vi "Diff Tool.vi"(10 "Reference":string, 11 "Target":string) -> (2 "Highlights":T1(array[cluster]), 3 "Result":string)   [LabVIEW 2020]
uses:
  d41eeba9-a009-4172-b538-d2f3e9e71bd9.vi
  <vilib>/Comparison/Less/Less Functor/Less Functor.lvclass
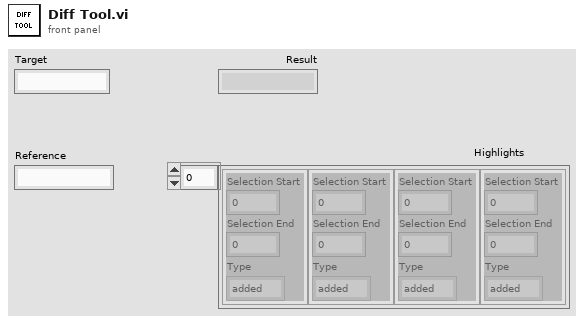
[diagram p1: front panel]
types:
  T1 = cluster{"Selection Start":u32, "Selection End":u32, "Type":enum16{"added", "missing"}}[]
  T2 = cluster{"Selection Start":u32, "Selection End":u32}[]
  T3 = cluster{"Index":i32, "String":string, "Type":enum16{"added", "missing"}}
  T4 = cluster{"Index":i32, "String":string, "Type":enum16{"added", "missing"}}[]
  T5 = cluster{"Selection Start":u32, "Selection End":u32, "Type":enum16{"added", "missing"}}
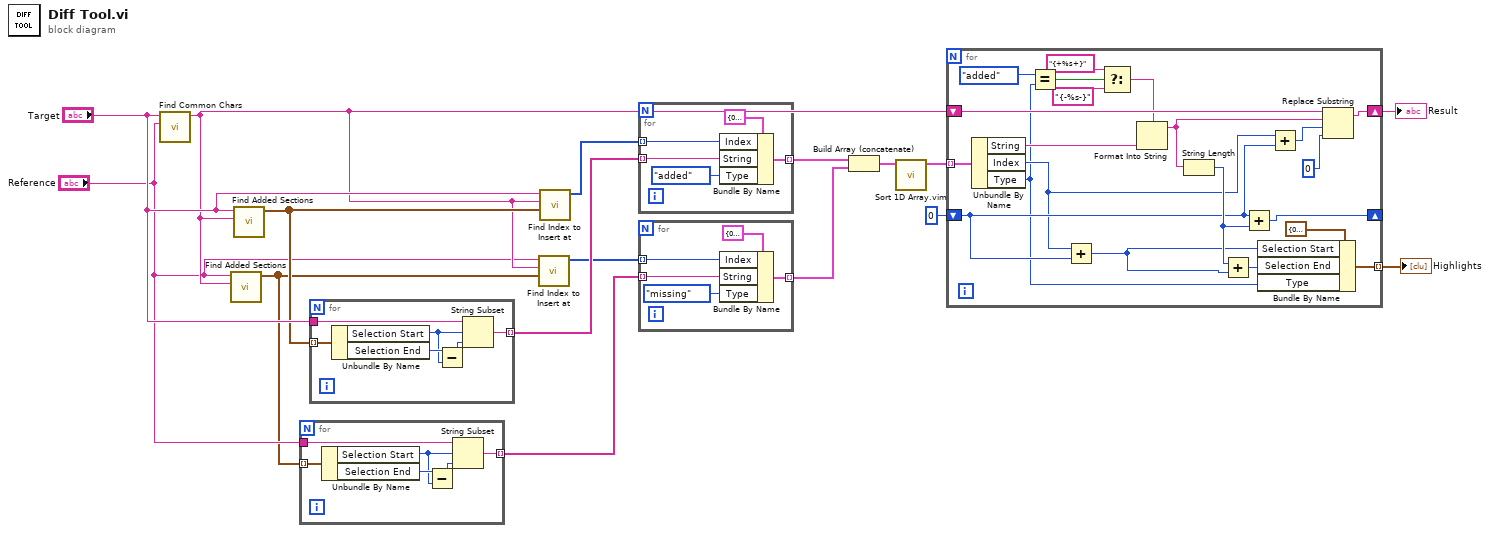
[diagram p0: block diagram]
diagram:
  n1 = call "Find Common Chars.vi"("Reference"="Reference", "Target"="Target") -> ("Common"=w13:string)  [unwired: 9 in]
  n2 = call "Find Added Sections.vi"("Reference"=w13, "Target"="Reference") -> ("Sections in Target"=w11:T2)  [unwired: 9 in]
  n3 = call "Find Added Sections.vi"("Reference"=w13, "Target"="Target") -> ("Sections in Target"=w15:T2)  [unwired: 9 in]
  n4 = for {
    tunnel: "Reference" -> [w22]
    tunnel: w11 -> [w21] mode=indexing
    tunnel: [w17] -> w5 mode=indexing
    n5 = Unbundle By Name(w21) -> ("Selection Start"=w19:u32, "Selection End"=w20:u32)
    n6 = Subtract(x=w20, y=w19) -> (x-y=w18:u32)
    n7 = String Subset(string=w22, offset (0)=w19, length (rest)=w18) -> (substring=w17:string)
  }
  n8 = for {
    tunnel: "Target" -> [w28]
    tunnel: w15 -> [w27] mode=indexing
    tunnel: [w23] -> w8 mode=indexing
    n9 = Unbundle By Name(w27) -> ("Selection Start"=w25:u32, "Selection End"=w26:u32)
    n10 = Subtract(x=w26, y=w25) -> (x-y=w24:u32)
    n11 = String Subset(string=w28, offset (0)=w25, length (rest)=w24) -> (substring=w23:string)
  }
  n12 = call "Find Index to Insert at.vi"("Sections in Target"=w11, "Reference"=w13, "Target"="Reference") -> ("Indices in Ref"=w6:i32[])  [unwired: 8 in]
  n13 = call "Find Index to Insert at.vi"("Sections in Target"=w15, "Reference"=w13, "Target"="Target") -> ("Indices in Ref"=w9:i32[])  [unwired: 8 in]
  n14 = for {
    tunnel: w9 -> [w32] mode=indexing
    tunnel: w8 -> [w31] mode=indexing
    tunnel: [w29] -> w7 mode=indexing
    n15 = Bundle By Name(cluster=T3 {"Index"=0, "String"="", "Type"=enum."added"}, "Index"=w32, "String"=w31, "Type"=enum16{"added", "missing"}."added") -> (w29:T3)
  }
  n16 = for {
    tunnel: w6 -> [w37] mode=indexing
    tunnel: w5 -> [w36] mode=indexing
    tunnel: [w34] -> w3 mode=indexing
    n17 = Bundle By Name(cluster=T3 {"Index"=0, "String"="", "Type"=enum."added"}, "Index"=w37, "String"=w36, "Type"=enum16{"added", "missing"}."missing") -> (w34:T3)
  }
  n18 = Build Array (concatenate)(w7, w3) -> (w4:T4)
  n19 = call "Sort 1D Array.vim"("unsorted array"=w4) -> ("sorted array"=w2:T4)  [unwired: 10 in]
  n20 = for {
    shift-right: [w58] -> w10
    shift-left: w13 -> [w59]
    tunnel: [w54] -> w14 mode=indexing
    shift-right: [w52] -> _
    shift-left: 0 -> [w48]
    tunnel: w2 -> [w47] mode=indexing
    n21 = Unbundle By Name(w47) -> ("String"=w45:string, "Index"=w46:i32, "Type"=w41:enum16{"added", "missing"})
    n22 = Equal?(x=enum16{"added", "missing"}."added", y=w41) -> (x = y?=w39:bool)
    n23 = Add(x=w46, y=w48) -> (x+y=w49:i32)
    n24 = Select(t="{+%s+}" ("format string"), s=w39, f="{-%s-}" ("format string")) -> (s? t:f=w42:string)
    n25 = Format Into String(format string=w42, w45) -> (resulting string=w56:string)  [unwired: 2 in, 1 out]
    n26 = String Length(string=w56) -> (length=w50:i32)
    n27 = Add(x=w50, y=w49) -> (x+y=w55:i32)
    n28 = Add(x=w48, y=w50) -> (x+y=w52:i32)
    n29 = Bundle By Name(cluster=T5 {"Selection Start"=0, "Selection End"=0, "Type"=enum."added"} ("Highlights"), "Selection Start"=w49, "Selection End"=w55, "Type"=w41) -> (w54:T5)
    n30 = Add(x=w46, y=w48) -> (x+y=w51:i32)
    n31 = Replace Substring(2:0 ("length (len. of substring)"), 3:w51, 4:w56, 5:w59) -> (1:w58:string)  [unwired: 1 out]
  }
  "Highlights" <- w14
  "Result" <- w10
